vi "GetButtonHelpText.vi"(0 "reference in":refnum<class "Graph.lvclass">, 2 "ButtonString":string, 5 "error in (no error)":errorcluster) -> (14 "reference out":refnum<class "Graph.lvclass">, 16 "HelpOut":T1, 19 "error out":errorcluster)   [LabVIEW 2016, in "Graph.lvclass"]
uses:
  <resource>/Framework/Providers/Open_GDS/UML/Graph_class/Graph.lvclass
  <resource>/Framework/Providers/Open_GDS/UML/ContextHelp/ContextHelp_ShowType.ctl
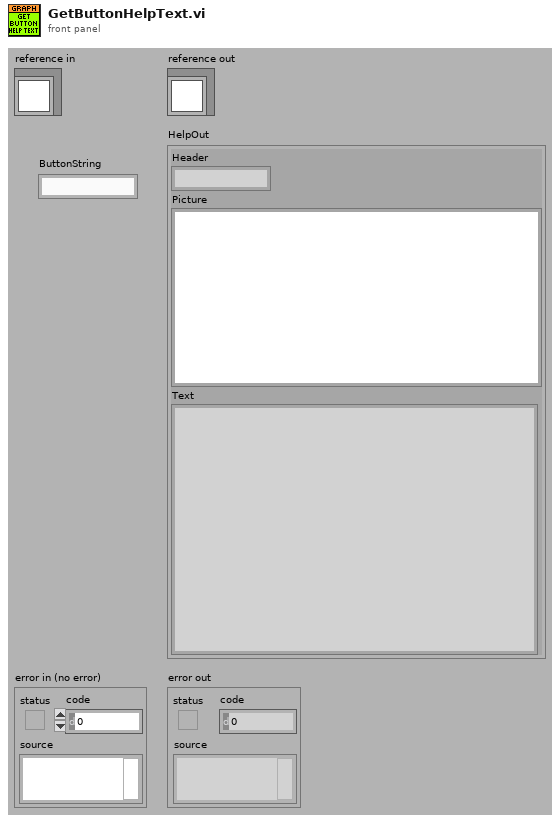
[diagram p1: front panel]
types:
  T1 = typedef "ContextHelp_ShowType.ctl" = cluster{"Header":string, "Picture":picture, "Text":string}
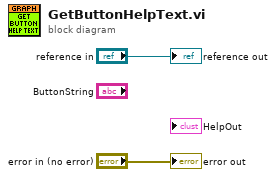
[diagram p0: block diagram]
diagram:
  "error out" <- "error in (no error)"
  "reference out" <- "reference in"
